vi "XY Graph Compute Plot Zero-Crossing Transform.vi"(8 "Error In":errorcluster, 9 "Shift":dbl, 10 "IRF Array in":dbl[](array[numeric]), 11 "t Array in":dbl[](array[numeric])) -> (0 "Error Out":errorcluster, 2 "ZC IRF Array out":dbl[](array[numeric]), 3 "t Array (dup) out":dbl[](array[numeric]))   [LabVIEW 2021, in "XY Graph Add-Ons.lvlib"]
uses:
  XY Graph Add-Ons.lvlib
panel:
  out "XY Graph":T1(graph)
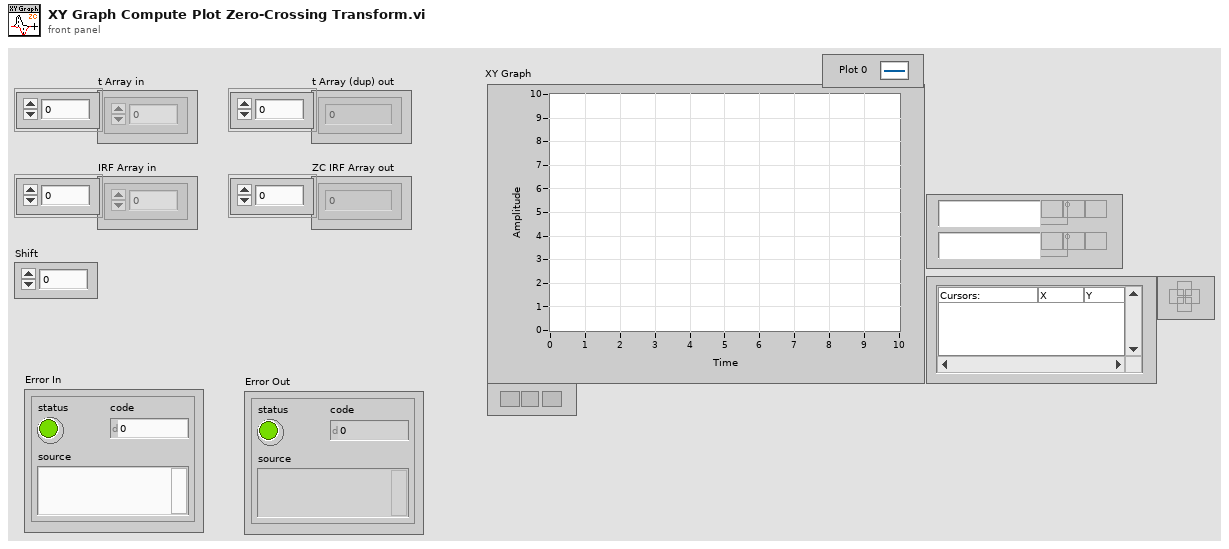
[diagram p1: front panel]
types:
  T1 = cluster{"t Array in":dbl[], "IRF Array in":dbl[]}
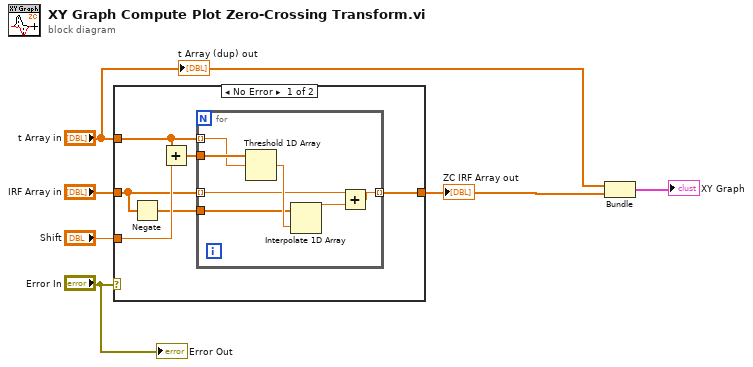
[diagram p0: block diagram]
diagram:
  n1 = case shown="No Error" "Error In" {
    tunnel: "t Array in" -> [w8 _]
    tunnel: "IRF Array in" -> [w11 w20]
    tunnel: [w10 w20] -> w4
    tunnel: "Shift" -> [w12 _]
    frame No Error {
      n2 = Negate(x=w11) -> (-x=w7:dbl[])
      n3 = Add(x=w8, y=w12) -> (x+y=w9:dbl[])
      n4 = for {
        tunnel: w9 -> [w17]
        tunnel: w8 -> [w13] mode=indexing
        tunnel: w7 -> [w18]
        tunnel: w11 -> [w16] mode=indexing
        tunnel: [w14] -> w10 mode=indexing
        n5 = Threshold 1D Array(2:w13, 3:w17) -> (0:w19:dbl)  [unwired: 1 in]
        n6 = Interpolate 1D Array(1:w19, 2:w18) -> (0:w15:dbl)
        n7 = Add(x=w16, y=w15) -> (x+y=w14:dbl)
      }
    }
    frame Error {
    }
  }
  "ZC IRF Array out" <- w4
  n8 = Bundle("t Array in"="t Array in", "IRF Array in"=w4) -> (→"XY Graph":T1)  [unwired: 1 in]
  "t Array (dup) out" <- "t Array in"
  "Error Out" <- "Error In"
